vi "VI Menu Example.vi"() -> ()   [LabVIEW 2016]
doc: "Demonstrates the Menu Strip type. Run the VI to see it's Runtime Menu replaced by the specified menu. Notice the shorcut key on the Exit Menu item.\n\nClick summarys show up in the history array. Click the \"Add Item\" to add a dummy item to the VI's menu."
uses:
  <vilib>/Utility/miscctls.llb/LVMenuShortCut.ctl
  <userlib>/_MGI/Menu Building/SelectionType/RadioSelection/MGI_RadioSelection.lvclass
  C:/Program Files (x86)/National Instruments/LabVIEW 2016/user.lib/_MGI/Menu Building/SelectionType/MGI_SelectionType.lvclass
  <userlib>/_MGI/Menu Building/SelectionType/CheckmarkSelection/MGI_CheckmarkSelection.lvclass
  <userlib>/_MGI/Menu Building/MenuItem/MenuSeparatorItem/MGI_MenuSeparatorItem.lvclass
  C:/Program Files (x86)/National Instruments/LabVIEW 2016/user.lib/_MGI/Menu Building/MenuItem/MGI_MenuItem.lvclass
  <userlib>/_MGI/Menu Building/MenuItem/VIItem/MGI_VIItem.lvclass
  <userlib>/_MGI/Menu Building/MenuTypes/Vi/MGI_VI.lvclass
  C:/Program Files (x86)/National Instruments/LabVIEW 2016/user.lib/_MGI/Menu Building/MenuTypes/MGI_Menu.lvclass
  <userlib>/_MGI/Menu Building/MenuItem/VIItem/VIItem.vi
  <userlib>/_MGI/Menu Building/MenuItem/MenuItem.vi
  <userlib>/_MGI/Menu Building/MenuItem/VIItem/Write short cut.vi
  <userlib>/_MGI/Menu Building/SelectionType/RadioSelection/RadioSelection.vi
  <userlib>/_MGI/Menu Building/MenuItem/Write Click By Default.vi
  <userlib>/_MGI/Menu Building/MenuItem/Write Sub-Menus.vi
  <userlib>/_MGI/Menu Building/MenuTypes/Vi/VI.vi
  <userlib>/_MGI/Menu Building/MenuItem/MenuSeparatorItem/MenuSeparatorItem.vi
  <userlib>/_MGI/Menu Building/SelectionType/CheckmarkSelection/CheckmarkSelection.vi
  <userlib>/_MGI/Menu Building/MenuTypes/Read Menu Items.vi
  <userlib>/_MGI/Menu Building/MenuItem/MGI_MenuItem.lvclass
  <userlib>/_MGI/Menu Building/MenuTypes/MGI_Menu.lvclass
  <userlib>/_MGI/Menu Building/SelectionType/MGI_SelectionType.lvclass
  <userlib>/_MGI/Menu Building/MenuItemStatusChange/MGI_MenuItemStatusChange.lvclass
panel:
  out "History":T1(array[cluster])
  in  "Add item":bool
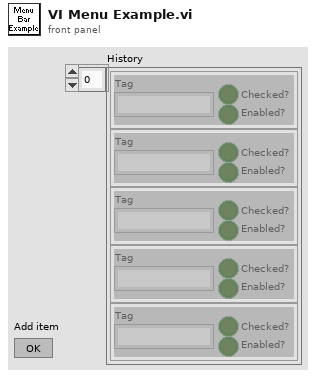
[diagram p1: front panel]
types:
  T1 = cluster{"Tag":string, "Checked?":bool, "Enabled?":bool}[]
  T2 = typedef "LVMenuShortCut.ctl" = cluster{"Include Shift Key?":bool, "Include Ctrl Key?":bool, "Shortcut Key":string}
  T3 = cluster{"Tag":string, "Checked?":bool, "Enabled?":bool}
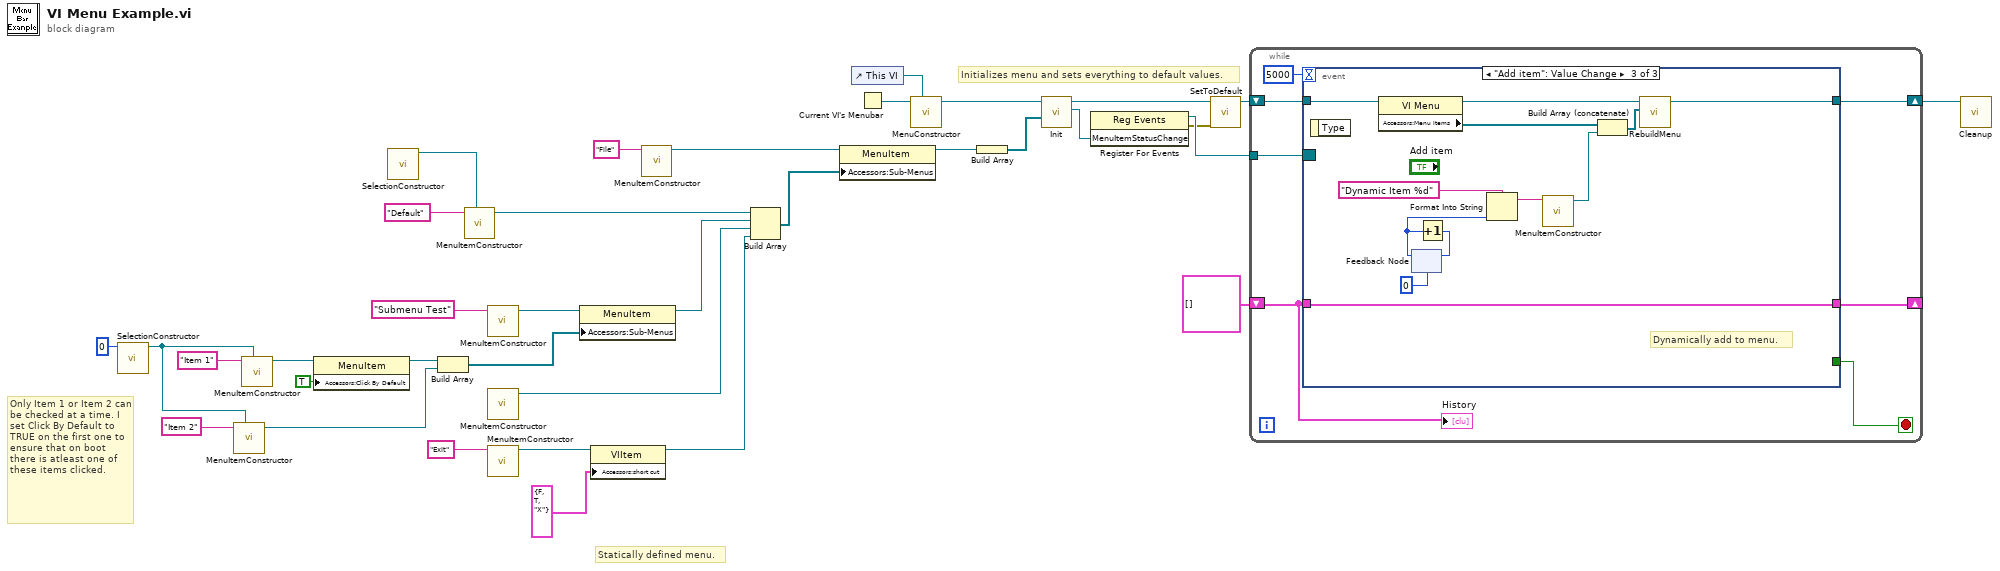
[diagram p0: block diagram]
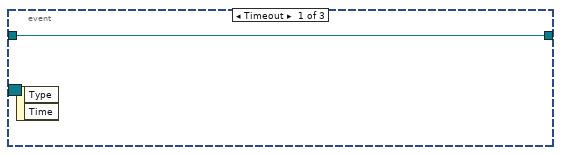
[diagram p2: hidden frame]
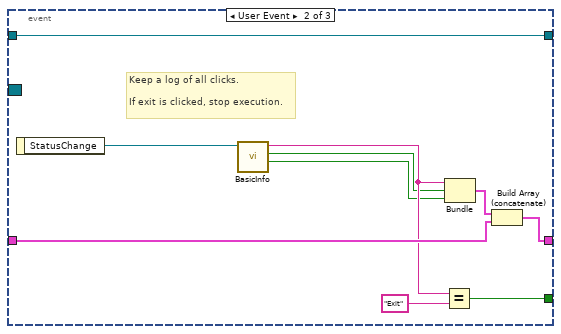
[diagram p3: hidden frame]
diagram:
  # "Initializes menu and sets everything to default values."
  # "Only Item 1 or Item 2 can be checked at a time. I set Click By Default to TRUE on the first one to ensure that on boot there is atleast one of these items clicked."
  # "Statically defined menu."
  n1 = call-poly <userlib>:"SelectionConstructor.vi"("Group"=u8 0) -> ("RadioSelection out"=w7:refnum<class "MGI_RadioSelection.lvclass">)  [unwired: 9 in, 1 out]
  n2 = call-poly <userlib>:"MenuItemConstructor.vi"("Selection Type"=w7, "Text"="Item 2") -> ("MenuItem"=w9:refnum<data-value>)  [unwired: 8 in, 1 out]
  n3 = call-poly <userlib>:"MenuItemConstructor.vi"("Selection Type"=w7, "Text"="Item 1") -> ("MenuItem"=w12:refnum<data-value>)  [unwired: 8 in, 1 out]
  n4 = property class="MenuItem"(reference=w12, "Accessors:Click By Default"=TRUE ("Click By Default")) -> (reference out=w5:refnum<data-value>)  [unwired: 1 in, 1 out]
  n5 = call-poly <userlib>:"SelectionConstructor.vi"() -> ("CheckmarkSelection out"=w6:refnum<class "MGI_CheckmarkSelection.lvclass">)  [unwired: 10 in, 1 out]
  n6 = Build Array(w5, w9) -> (w29:refnum<data-value>[])
  n7 = call-poly <userlib>:"MenuItemConstructor.vi"("Selection Type"=w6, "Text"="Default") -> ("MenuItem"=w19:refnum<data-value>)  [unwired: 8 in, 1 out]
  n8 = call-poly <userlib>:"MenuItemConstructor.vi"("Text"="Submenu Test") -> ("MenuItem"=w16:refnum<data-value>)  [unwired: 9 in, 1 out]
  n9 = call-poly <userlib>:"MenuItemConstructor.vi"() -> ("MenuSeparatorItem"=w15:refnum<data-value>)  [unwired: 10 in, 1 out]
  n10 = call-poly <userlib>:"MenuItemConstructor.vi"("Text"="Exit") -> ("VIItem Item"=w14:refnum<data-value>)  [unwired: 9 in, 1 out]
  n11 = property class="MenuItem"(reference=w16, "Accessors:Sub-Menus"=w29) -> (reference out=w28:refnum<data-value>)  [unwired: 1 in, 1 out]
  n12 = property class="VIItem"(reference=w14, "Accessors:short cut"=T2 {"Include Shift Key?"=FALSE, "Include Ctrl Key?"=TRUE, "Shortcut Key"="X"} ("short cut")) -> (reference out=w30:refnum<data-value>)  [unwired: 1 in, 1 out]
  n13 = call-poly <userlib>:"MenuItemConstructor.vi"("Text"="File") -> ("MenuItem"=w21:refnum<data-value>)  [unwired: 9 in, 1 out]
  n14 = Build Array(w19, w28, w15, w30) -> (w27:refnum<data-value>[])
  n15 = property class="MenuItem"(reference=w21, "Accessors:Sub-Menus"=w27) -> (reference out=w26:refnum<data-value>)  [unwired: 1 in, 1 out]
  n16 = control-ref of="This VI"() -> (w22:refnum<vi>)
  n17 = Current VI's Menubar() -> (w23:refnum<k9>)
  n18 = call-poly <userlib>:"MenuConstructor.vi"("Menu VI"=w22, "menu reference"=w23) -> ("VI"=w24:refnum<class "MGI_VI.lvclass">)  [unwired: 8 in, 1 out]
  n19 = Build Array(w26) -> (w25:refnum<data-value>[])
  n20 = call-dynamic "Init.vi"("Menu Items"=w25, "Menu in"=w24) -> ("MenuItemStatusChange"=w35:refnum<user-event>, "Menu out"=w33:refnum<class "MGI_VI.lvclass">)  [unwired: 7 in, 1 out]
  n21 = register-events(w35) -> (reference out=w34:refnum<event-registration>, error out=w31:errorcluster)  [unwired: 2 in]
  n22 = call-dynamic "SetToDefault.vi"("error in (no error)"=w31, "Menu in"=w33) -> ("Menu out"=w32:refnum<class "MGI_VI.lvclass">)  [unwired: 8 in, 1 out]
  n23 = while {
    tunnel: w34 -> [w42]
    shift-right: [w40] -> _
    shift-left: T1 [] -> [w36]
    shift-right: [w37] -> w3
    shift-left: w32 -> [w38]
    stop <- w41 stop-if-true
    n24 = event shown="[2] \"Add item\": Value Change" {
      selector: w42 -> [_ _ _]
      dyn-events: _ -> [_ _ _]
      timeout: 5000 -> [_ _ _]
      tunnel: [_ w52 _] -> w41
      tunnel: [_ w51 w59] -> w40
      tunnel: w36 -> [_ w50 w59]
      tunnel: w38 -> [w43 w49 w65]
      tunnel: [w43 w49 w64] -> w37
      event Timeout {
        n25 = event-data() -> ()  [unwired: 1 in, 2 out]
      }
      event User Event {
        # "Keep a log of all clicks.\n\nIf exit is clicked, stop execution."
        n26 = event-data() -> ("StatusChange"=w48:refnum<class "MGI_MenuItemStatusChange.lvclass">)  [unwired: 1 in]
        n27 = call <userlib>:"BasicInfo.vi"("MGI_MenuItemStatusChange in"=w48) -> ("Enabled?"=w46:bool, "Checked?"=w45:bool, "Tag"=w47:string)  [unwired: 7 in, 1 out]
        n28 = Equal?(x=w47, y="Exit") -> (x = y?=w52:bool)
        n29 = Bundle("Tag"=w47, "Checked?"=w45, "Enabled?"=w46) -> (w44:T3)  [unwired: 1 in]
        n30 = Build Array (concatenate)(w44, w50) -> (w51:T1)
      }
      event "Add item": Value Change {
        # "Dynamically add to menu."
        n31 = event-data() -> ()  [unwired: 1 in, 1 out]
        n32 = property class="VI Menu"(reference=w65) -> (reference out=w63:refnum<class "MGI_VI.lvclass">, "Accessors:Menu Items"=w62:refnum<data-value>[])  [unwired: 1 in, 1 out]
        n33 = feedback #1(0) -> (w56:i32)
        n34 = Increment(x=w56) -> (x+1=w55:i32)
        n35 = feedback-in #1(w55) -> ()
        n36 = Format Into String(format string="Dynamic Item %d" ("Text"), w56) -> (resulting string=w54:string)  [unwired: 2 in, 1 out]
        n37 = call-poly <userlib>:"MenuItemConstructor.vi"("Text"=w54) -> ("MenuItem"=w60:refnum<data-value>)  [unwired: 9 in, 1 out]
        n38 = Build Array (concatenate)(w62, w60) -> (w61:refnum<data-value>[])
        n39 = call <userlib>:"RebuildMenu.vi"("New Menu Items"=w61, "Menu in"=w63) -> ("Menu out"=w64:refnum<class "MGI_VI.lvclass">)  [unwired: 8 in, 1 out]
      }
    }
    "History" <- w36
  }
  n40 = call-dynamic "Cleanup.vi"("VI"=w3) -> ()  [unwired: 10 in, 1 out]
